vi "FTW-Actor-Destroy.vi"(0 "FTW Actor Instance":refnum<class "FTW-Actor-Instance.lvclass">, 11 "error in":errorcluster) -> (6 "Remaining Jobs":string, 15 "error out":errorcluster)   [LabVIEW 2015, in "FTW-Actor-Instance.lvclass"]
uses:
  FTW-Actor-Instance.lvclass
  scheduler/FTW-Scheduler.lvclass
panel:
  # "Inputs"
  # "Outputs"
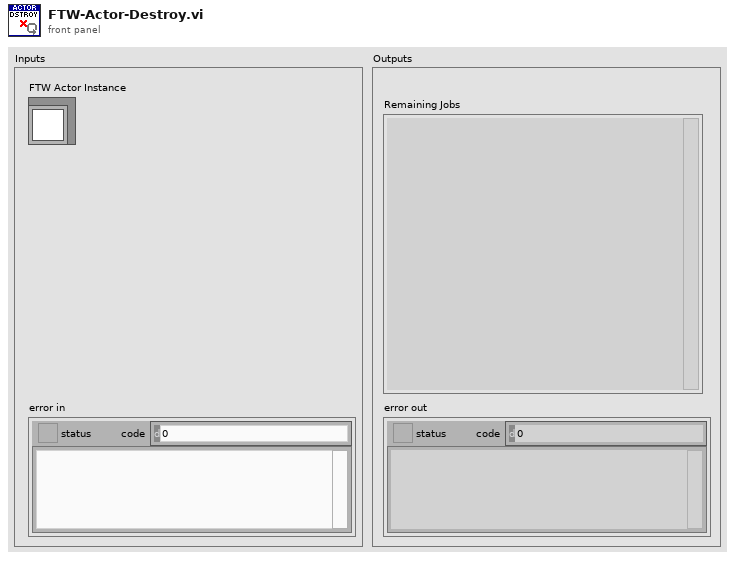
[diagram p1: front panel]
types:
  T1 = typedef "FTW-Type-Actor-Inbox.ctl" = refnum<data-value>
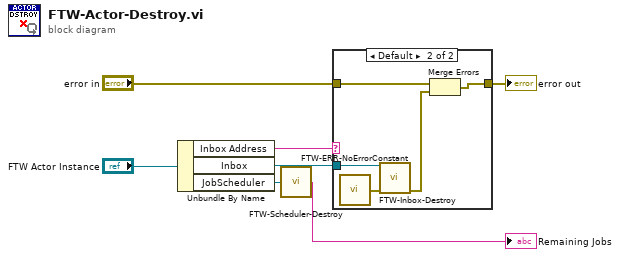
[diagram p0: block diagram]
diagram:
  n1 = Unbundle By Name("FTW Actor Instance") -> ("Inbox Address"=w6:string, "Inbox"=w7:T1, "JobScheduler"=w4:refnum<class "FTW-Scheduler.lvclass">)
  n2 = call "FTW-Scheduler-Destroy.vi"("FTW Job Scheduler"=w4) -> ("Remaining Jobs"=→"Remaining Jobs":string)
  n3 = case shown="Default" w6 {
    tunnel: w7 -> [_ w13]
    tunnel: [w8 w9] -> w3
    tunnel: "error in" -> [w8 w12]
    frame "" {
    }
    frame Default {
      n4 = call "FTW-ERR-NoErrorConstant.vi"() -> ("no error"=w11:errorcluster)
      n5 = call "FTW-Inbox-Destroy.vi"("FTW Inbox"=w13, "error in"=w11) -> ("error out"=w10:errorcluster)  [unwired: 13 in]
      n6 = Merge Errors(w12, w10) -> (w9:errorcluster)
    }
  }
  "error out" <- w3
